vi "generate_trajectory.vi"(8 "error in (no error)":errorcluster, 11 "DL090202ScanHead in":refnum<class "ScanHeadDL090202.lvclass">) -> (0 "error out":errorcluster, 3 "DL090202ScanHead out":refnum<class "ScanHeadDL090202.lvclass">)   [LabVIEW 2010, in "ScanHeadDL090202.lvclass"]
uses:
  ScanHeadDL090202.lvclass
  Trajectory/TrajectoryDL091126GenericVoxel/TrajectoryDL091126GenericVoxel/TrajectoryDL091126GenericVoxel.lvclass
  common/enumerations/functional_global_action_enum.ctl
  Trajectory/GenericTrajectory/GenericTrajectory/GenericTrajectory.lvclass
  common/classes/ErrorController/ErrorController/ErrorController.lvclass
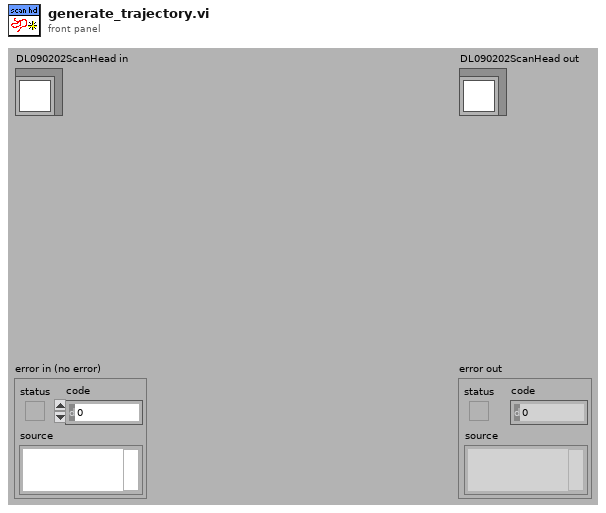
[diagram p1: front panel]
types:
  T1 = typedef "functional_global_action_enum.ctl" = enum16{"get", "set", "reset"}
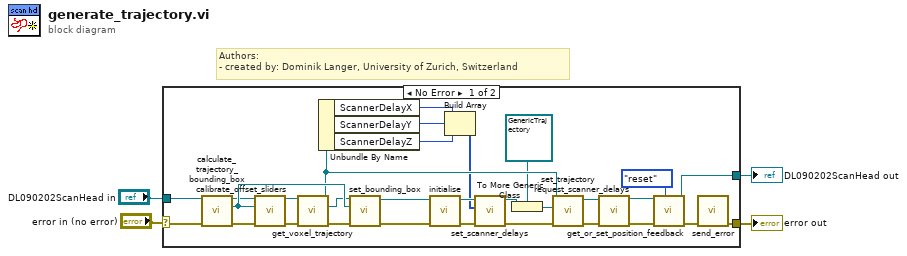
[diagram p0: block diagram]
diagram:
  # "Authors: \n- created by: Dominik Langer, University of Zurich, Switzerland"
  n1 = case shown="No Error" "error in (no error)" {
    selector: "error in (no error)" -> [w31 w36]
    tunnel: [w7 w36] -> w3
    tunnel: [w19 w35] -> w1
    tunnel: "DL090202ScanHead in" -> [w30 w35]
    frame No Error {
      n2 = call-dynamic "calculate_trajectory_bounding_box.vi"("error in (no error)"=w31, "DL090202ScanHead in"=w30) -> ("error out"=w32:errorcluster, "bounding box"=w34:refnum<class "Box.lvclass">, "DL090202ScanHead out"=w33:refnum<class "ScanHeadDL090202.lvclass">)  [unwired: 7 out]
      n3 = call-dynamic "calibrate_offset_sliders.vi"("error in (no error)"=w32, "trajectory bounding box"=w34, "DL090202ScanHead in"=w33) -> ("error out"=w29:errorcluster, "DL090202ScanHead out"=w28:refnum<class "ScanHeadDL090202.lvclass">)  [unwired: 7 out]
      n4 = call-dynamic "get_voxel_trajectory.vi"("error in (no error)"=w29, "ScanHeadDL090202 in"=w28) -> ("error out"=w26:errorcluster, "trajectory"=w27:refnum<class "TrajectoryDL091126GenericVoxel.lvclass">, "ScanHeadDL090202 out"=w25:refnum<class "ScanHeadDL090202.lvclass">)  [unwired: 7 in]
      n5 = Unbundle By Name(w25) -> ("ScannerDelayX"=w10:i32, "ScannerDelayY"=w11:i32, "ScannerDelayZ"=w12:i32)
      n6 = call-dynamic "set_bounding_box.vi"("error in (no error)"=w26, "Box.lvclass"=w34, "GenericTrajectory in"=w27) -> ("error out"=w6:errorcluster, "GenericTrajectory out"=w5:refnum<class "TrajectoryDL091126GenericVoxel.lvclass">)  [unwired: 7 out]
      n7 = call-dynamic "initialise.vi"("error in (no error)"=w6, "GenericTrajectory in"=w5) -> ("error out"=w18:errorcluster, "GenericTrajectory out"=w17:refnum<class "TrajectoryDL091126GenericVoxel.lvclass">)  [unwired: 8 out]
      n8 = Build Array(w10, w11, w12) -> (w9:i32[])
      n9 = call-dynamic "set_scanner_delays.vi"("error in (no error)"=w18, "scanner delays"=w9, "TrajectoryDL091126GenericVoxel in"=w17) -> ("error out"=w15:errorcluster, "TrajectoryDL091126GenericVoxel out"=w16:refnum<class "TrajectoryDL091126GenericVoxel.lvclass">)  [unwired: 7 in]
      n10 = To More Generic Class(target class=refnum<class "GenericTrajectory.lvclass"> refnum ("trajectory"), reference=w16) -> (generic class reference=w13:refnum<class "GenericTrajectory.lvclass">)
      n11 = call-dynamic "set_trajectory.vi"("error in (no error)"=w15, "trajectory"=w13, "GenericScanHead.lvclass in"=w25) -> ("error out"=w24:errorcluster, "GenericScanHead.lvclass out"=w23:refnum<class "ScanHeadDL090202.lvclass">)  [unwired: 7 out]
      n12 = call-dynamic "request_scanner_delays.vi"("error in (no error)"=w24, "ScanHeadDL090202 in"=w23) -> ("error out"=w22:errorcluster, "ScanHeadDL090202 out"=w21:refnum<class "ScanHeadDL090202.lvclass">)  [unwired: 8 in]
      n13 = call-dynamic "get_or_set_position_feedback.vi"("action"=functional_global_action_enum."reset", "error in (no error)"=w22, "ScanHeadDL090202 in"=w21) -> ("error out"=w8:errorcluster, "ScanHeadDL090202 out"=w19:refnum<class "ScanHeadDL090202.lvclass">)  [unwired: 6 in, 1 out]
      n14 = call "send_error.vi"("error in (no error)"=w8) -> ("error out"=w7:errorcluster)  [unwired: 10 in]
    }
    frame Error {
    }
  }
  "error out" <- w3
  "DL090202ScanHead out" <- w1
